vi "Disable_all_channels_ASIC.vi"(6 "CompBuf_en_b":bool=TRUE, 7 "Att_en_b":bool=TRUE, 8 "error in":errorcluster, 9 "id_in":i32, 10 "Clip_en_b":bool=TRUE, 11 "connection ID":refnum<k5>) -> (0 "error out":errorcluster, 1 "id_out":i32, 3 "connection ID out":refnum<k5>)   [LabVIEW 2009]
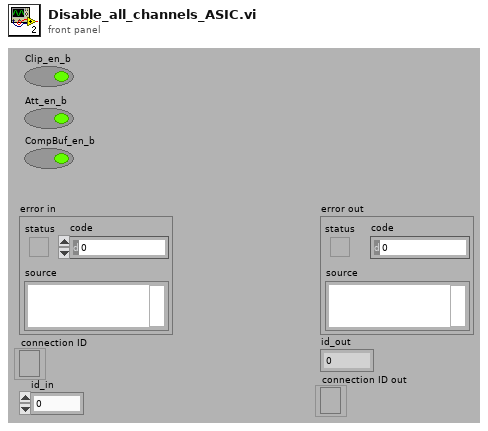
[diagram p1: front panel]
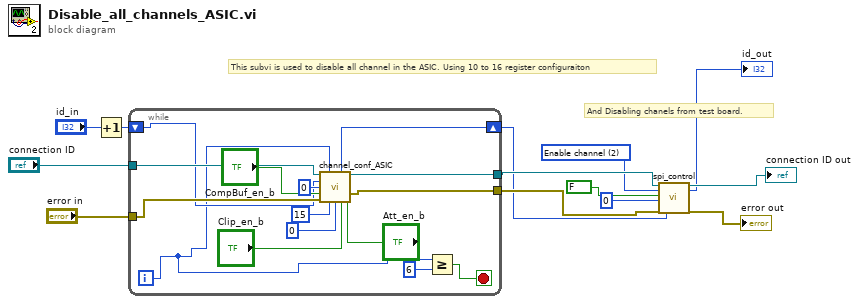
[diagram p0: block diagram]
diagram:
  w3 = u16 2 items=["Attenuation", "Clipping", "Enable channel", "Delay line", "ASIC"] ("Device")
  # "And Disabling chanels from test board."
  # "This subvi is used to disable all channel in the ASIC. Using 10 to 16 register configuraiton"
  n1 = Increment(x="id_in") -> (x+1=w11:i32)
  n2 = while {
    tunnel: "error in" -> [w26]
    shift-right: [w19] -> w4
    shift-left: w11 -> [w20]
    tunnel: "connection ID" -> [w25]
    tunnel: [w24] -> w9
    tunnel: [w23] -> w8
    i -> [w18]
    stop <- w28 stop-if-true
    n3 = call "channel_conf_ASIC.vi"("connection ID"=w25, "Ring"=w18, "Id in"=w20, "Clip_sel_b"=u32 0, "CompBuf_en_b"="CompBuf_en_b", "error out"=w26, "Att gain"=u32 15, "Ib_ClipVb"=u32 0, "Clip_en_b"="Clip_en_b", "Att_en_b"="Att_en_b") -> ("Id out"=w19:i32, "connection ID out"=w24:refnum<k5>, "error out 2"=w23:errorcluster)  [unwired: 1 in, 2 out]
    n4 = Greater Or Equal?(x=w18, y=6) -> (x >= y?=w28:bool)
  }
  n5 = call "spi_control.vi"("connection ID"=w9, "Device"=w3, "Read/#write"=FALSE, "Data"=0, "error out 3"=w8, "Id in"=w4) -> ("connection ID out"=→"connection ID out":refnum<k5>, "Id out"=→"id_out":i32, "error out 2"=→"error out":errorcluster)  [unwired: 6 in, 5 out]
